vi "4155C QSCV Config SMUs v3.0.vi"(0 "VISA resource name in":refnum<visa-resource-name>, 1 "QSCV - Probe 4":u32(ring)=3 items=["SMU1  ", "SMU2  ", "SMU3  ", "SMU4  ", "SMU5  ", "SMU6  ", "VSU1  ", "VSU2  "], 2 "Gate mode":u16(ring) items=["Auto", "Limited", "Fixed"], 3 "Gate Range":u8(slide)=6 max=11 scale=0.0..11.0, 5 "QSCV - Source/Common":u32(ring) items=["SMU1  ", "SMU2  ", "SMU3  ", "SMU4  ", "SMU5  ", "SMU6  ", "VSU1  ", "VSU2  "], 7 "QSCV - Drain":u32(ring)=1 items=["SMU1  ", "SMU2  ", "SMU3  ", "SMU4  ", "SMU5  ", "SMU6  ", "VSU1  ", "VSU2  "], 9 "QSCV - Gate":u32(ring)=2 items=["SMU1  ", "SMU2  ", "SMU3  ", "SMU4  ", "SMU5  ", "SMU6  ", "VSU1  ", "VSU2  "], 11 "error in (no error)":errorcluster, 13 "Source/drain mode":u16(ring) items=["Auto", "Limited", "Fixed"], 14 "Source/drain Range":u8(slide)=6 max=11 scale=0.0..11.0) -> (4 "VISA Resource Name out":refnum<visa-resource-name>, 15 "error out":errorcluster)   [LabVIEW 2016]
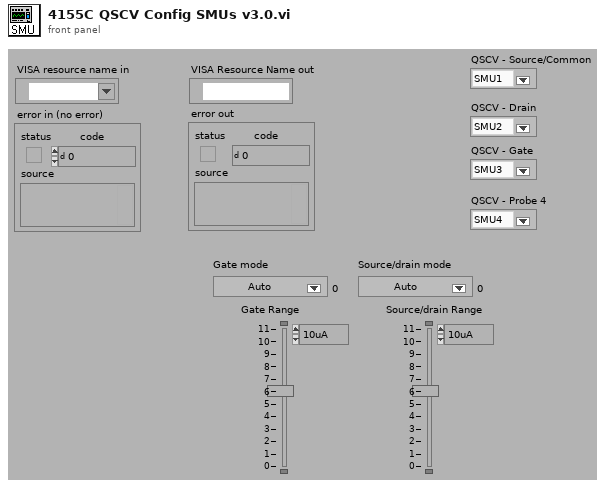
[diagram p1: front panel]
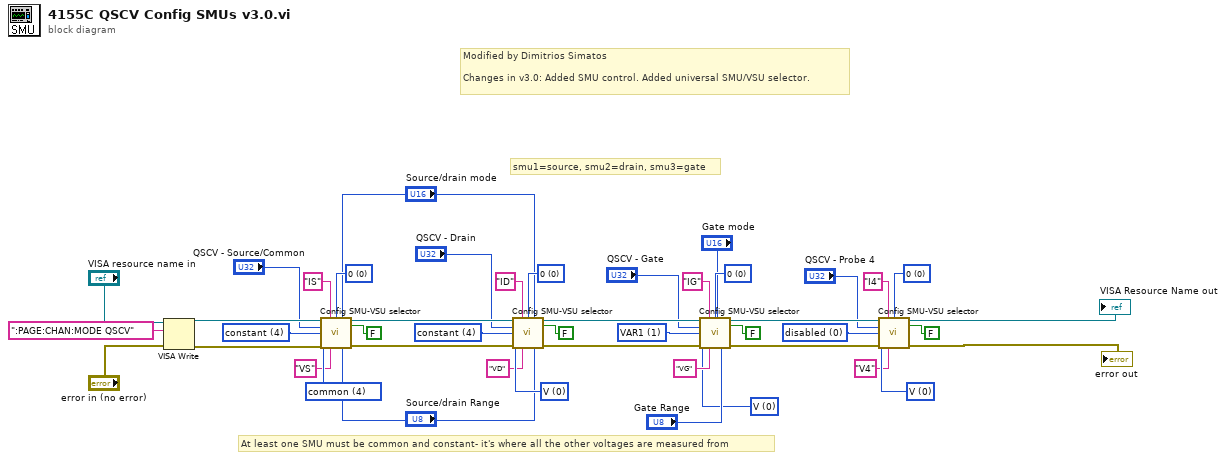
[diagram p0: block diagram]
diagram:
  w12 = u32 0 items=["V  ", "I  ", "V pulse  ", "I pulse  ", "  common  "] ("mode")
  w25 = u32 0 items=["V  ", "I  ", "V pulse  ", "I pulse  ", "  common  "] ("mode")
  w26 = u32 0 items=["0  ", "10K Ohms  ", "100K Ohms  ", "1M Ohms  "] ("series resistance *")
  w28 = u32 0 items=["disabled  ", "VAR1  ", "VAR2  ", "VAR1'  ", "constant  "] ("function")
  w31 = u32 0 items=["0  ", "10K Ohms  ", "100K Ohms  ", "1M Ohms  "] ("series resistance *")
  w33 = u32 1 items=["disabled  ", "VAR1  ", "VAR2  ", "VAR1'  ", "constant  "] ("function")
  w36 = u32 0 items=["V  ", "I  ", "V pulse  ", "I pulse  ", "  common  "] ("mode")
  w37 = u32 0 items=["0  ", "10K Ohms  ", "100K Ohms  ", "1M Ohms  "] ("series resistance *")
  w39 = u32 4 items=["disabled  ", "VAR1  ", "VAR2  ", "VAR1'  ", "constant  "] ("function")
  w42 = u32 4 items=["V  ", "I  ", "V pulse  ", "I pulse  ", "  common  "] ("mode")
  w43 = u32 0 items=["0  ", "10K Ohms  ", "100K Ohms  ", "1M Ohms  "] ("series resistance *")
  w45 = u32 4 items=["disabled  ", "VAR1  ", "VAR2  ", "VAR1'  ", "constant  "] ("function")
  # "Modified by Dimitrios Simatos\n\nChanges in v3.0: Added SMU control. Added universal SMU/VSU selector."
  # "smu1=source, smu2=drain, smu3=gate"
  # "At least one SMU must be common and constant- it's where all the other voltages are measured from"
  n1 = VISA Write(VISA resource name="VISA resource name in", write buffer=":PAGE:CHAN:MODE QSCV" ("write buffer (\"\")"), error in (no error)="error in (no error)") -> (VISA resource name out=w10:refnum<visa-resource-name>, error out=w11:errorcluster)  [unwired: 1 out]
  n2 = call "Config SMU-VSU selector.vi"("VISA session"=w10, "I name (max 6 chars)"="IS", "standby"=FALSE, "Range mode"="Source/drain mode", "unit to configure"="QSCV - Source/Common", "function"=w45, "mode"=w42, "error in (no error)"=w11, "V name (max 6 chars)"="VS", "series resistance *"=w43, "Range"="Source/drain Range") -> ("dup VISA resource name"=w22:refnum<visa-resource-name>, "error out"=w21:errorcluster)  [unwired: 1 in, 2 out]
  n3 = call "Config SMU-VSU selector.vi"("VISA session"=w22, "I name (max 6 chars)"="ID", "standby"=FALSE, "Range mode"="Source/drain mode", "unit to configure"="QSCV - Drain", "function"=w39, "mode"=w36, "error in (no error)"=w21, "V name (max 6 chars)"="VD", "series resistance *"=w37, "Range"="Source/drain Range") -> ("dup VISA resource name"=w19:refnum<visa-resource-name>, "error out"=w20:errorcluster)  [unwired: 1 in, 2 out]
  n4 = call "Config SMU-VSU selector.vi"("VISA session"=w19, "I name (max 6 chars)"="IG", "standby"=FALSE, "Range mode"="Gate mode", "unit to configure"="QSCV - Gate", "function"=w33, "mode"=w12, "error in (no error)"=w20, "V name (max 6 chars)"="VG", "series resistance *"=w31, "Range"="Gate Range") -> ("dup VISA resource name"=w18:refnum<visa-resource-name>, "error out"=w17:errorcluster)  [unwired: 1 in, 2 out]
  n5 = call "Config SMU-VSU selector.vi"("VISA session"=w18, "I name (max 6 chars)"="I4", "standby"=FALSE, "unit to configure"="QSCV - Probe 4", "function"=w28, "mode"=w25, "error in (no error)"=w17, "V name (max 6 chars)"="V4", "series resistance *"=w26) -> ("dup VISA resource name"=→"VISA Resource Name out":refnum<visa-resource-name>, "error out"=→"error out":errorcluster)  [unwired: 3 in, 2 out]
